vi "Set Pending Transfers.vi"(8 "error in":errorcluster, 10 "Pending Transfers":refnum<data-value>, 11 "SDO Manager Worker in":refnum<class "SDO Manager Worker.lvclass">) -> (0 "error out":errorcluster, 3 "SDO Manager Worker out":refnum<class "SDO Manager Worker.lvclass">)   [LabVIEW 2020, in "SDO Manager.lvlib" / "SDO Manager Worker.lvclass"]
uses:
  SDO Manager Worker.lvclass
  SDO Transfer/SDO Transfer.lvclass
  SDO Manager Worker.lvclass/SDO Manager Worker.ctl
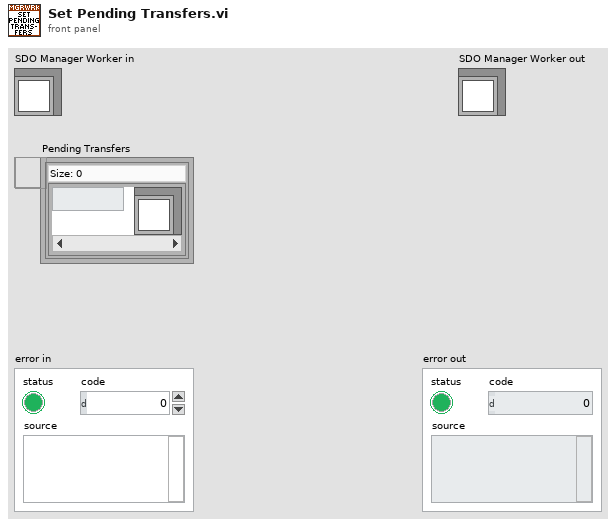
[diagram p1: front panel]
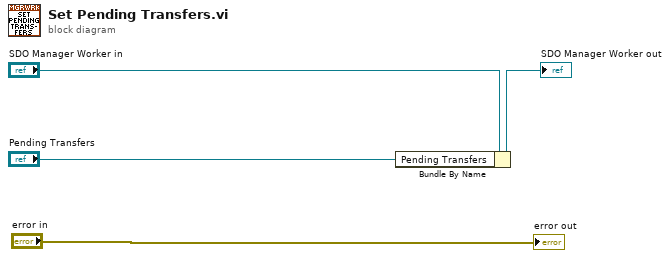
[diagram p0: block diagram]
diagram:
  n1 = Bundle By Name(cluster="SDO Manager Worker in", "Pending Transfers"="Pending Transfers") -> (→"SDO Manager Worker out":refnum<class "SDO Manager Worker.lvclass">)
  "error out" <- "error in"
